vi "Write Camera SN U64.vi"(8 "error in (no error)":errorcluster, 10 "Camera SN U64":u64, 11 "DAQcamera in":refnum<class "DAQcamera.lvclass">) -> (0 "error out":errorcluster, 3 "DAQcamera out":refnum<class "DAQcamera.lvclass">)   [LabVIEW 2016, in "DAQcamera.lvclass"]
uses:
  DAQcamera.lvclass
  DAQcamera.lvclass/DAQcamera.ctl
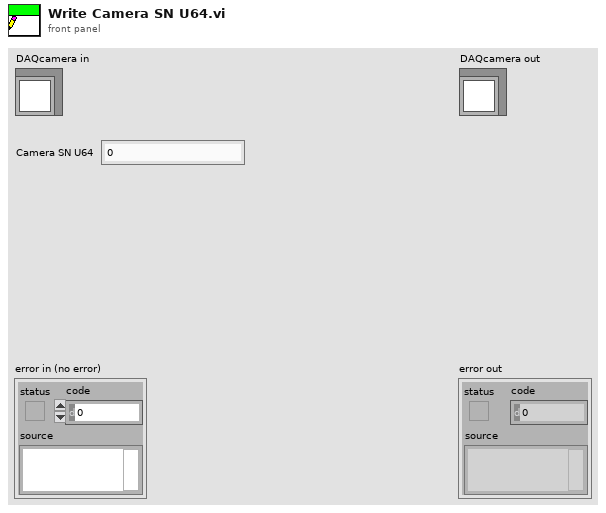
[diagram p1: front panel]
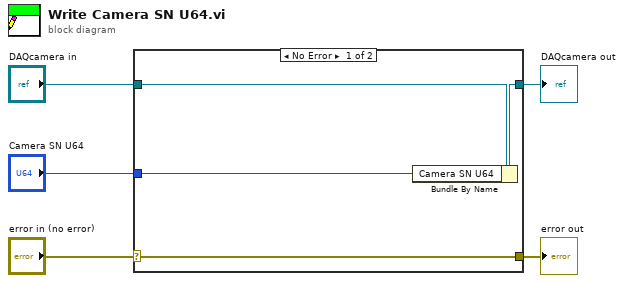
[diagram p0: block diagram]
diagram:
  n1 = case shown="No Error" "error in (no error)" {
    selector: "error in (no error)" -> [w9 w10]
    tunnel: [w9 w10] -> w4
    tunnel: [w7 w11] -> w2
    tunnel: "DAQcamera in" -> [w8 w11]
    tunnel: "Camera SN U64" -> [w6 _]
    frame No Error {
      n2 = Bundle By Name(cluster=w8, "Camera SN U64"=w6) -> (w7:refnum<class "DAQcamera.lvclass">)
    }
    frame Error {
    }
  }
  "error out" <- w4
  "DAQcamera out" <- w2
